vi "K-Means Clusters 1D.vi"() -> ()   [LabVIEW 2018]
uses:
  <vilib>/Analysis/5stat.llb/RMS (DBL).vi
  <vilib>/Analysis/baseanly.llb/Mean (DBL).vi
  <vilib>/Analysis/NI_AALBase.lvlib
  <vilib>/Analysis/NI_AALPro.lvlib
panel:
  out "Statistics":cluster{"mean":dbl, "rms":dbl, "median":dbl}[](array[cluster])
  out "Iteration":i32
  in  "Abs Max":dbl=100.0
  in  "Abs Min":dbl=-100.0
  in  "Normalize":T1(ring)
  out "K-Means Clusters":cluster{dbl[]}[](array[cluster])
  out "K-Means Graph":cluster{dbl[]}[](graph)
  in  "Num of Clusters (5)":i32=5
  in  "Data Set":dbl[](array[numeric])=[11.0, 12.0, 13.0, 21.0, 22.0, 23.0, 31.0, 32.0, 33.0, 41.0, 42.0, 43.0, 51.0, 52.0, 53.0, 16.0, 17.0, 18.0, 16.0]
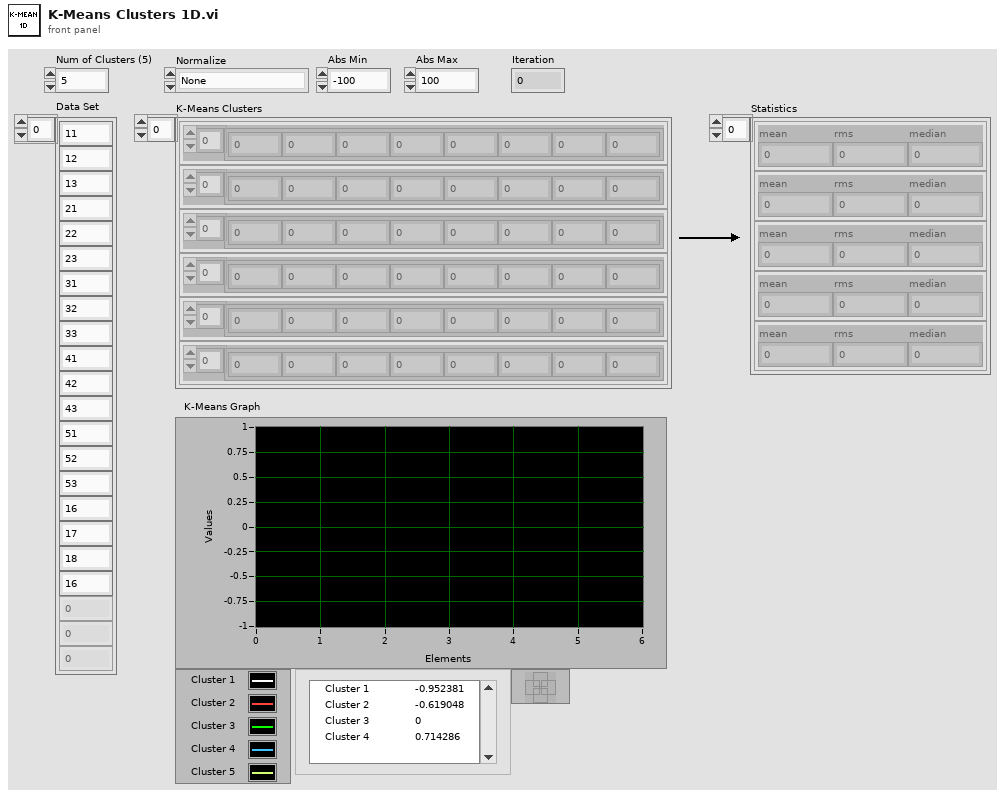
[diagram p1: front panel]
types:
  T1 = enum16{"None", "Data Set Min..Max -> 0..1", "Data Set Min..Max -> -1..1", "Absolute Min..Max -> 0..1", "Absolute Min..Max -> -1..1"}
  T2 = cluster{"mean":dbl, "rms value":dbl, "median":dbl}
  T3 = cluster{"Name":string, "Color":u32, "Style":u8, "Point Style":u8, "Name Visible":bool, "Allow Drag":bool, "Cursor Mode":u32, "Plot":i32, "Index":i32, "Position":cluster{"X":dbl, "Y":dbl}, "X Scale":u32, "Y Scale":u32, "Watch Plots":i32[], "Watch All Plots":bool, "Plot Area":i32, "Label Offset":cluster{"X":dbl, "Y":dbl}}
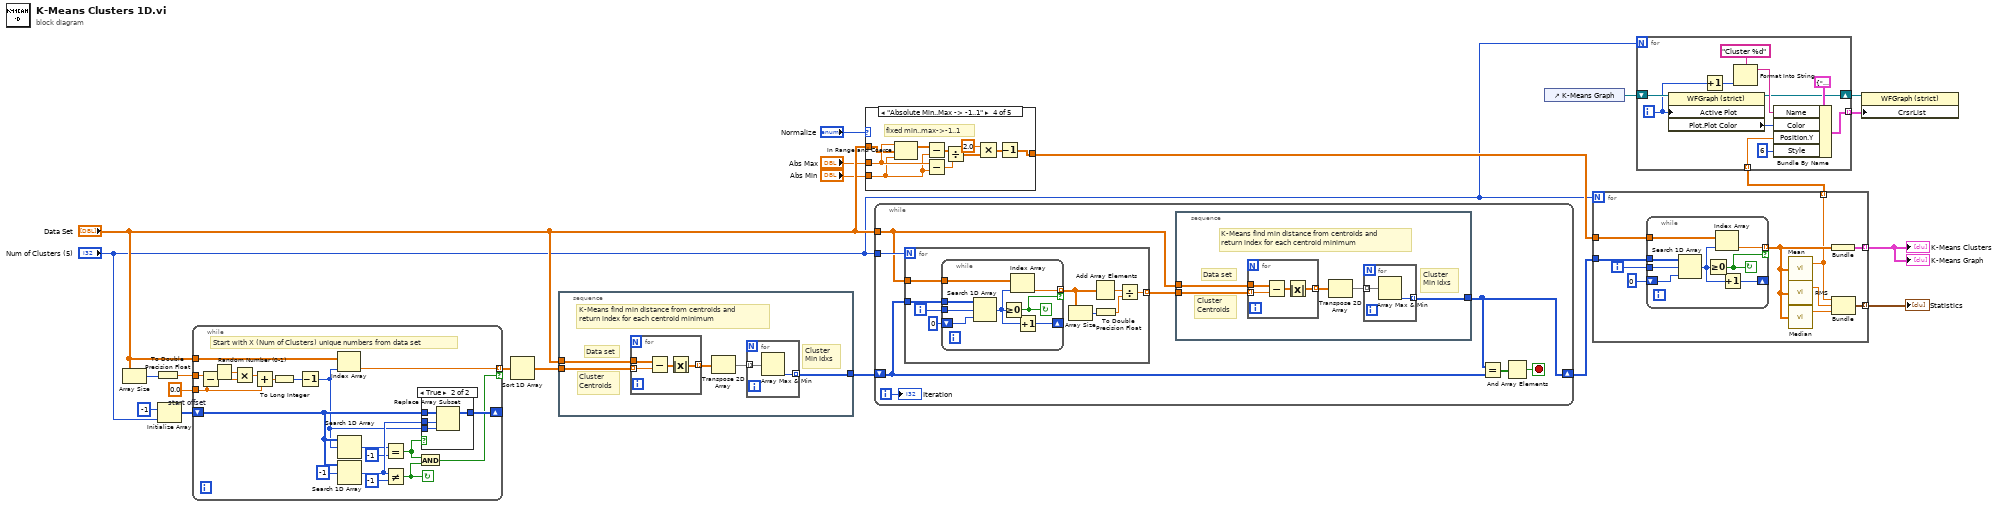
[diagram p0: block diagram]
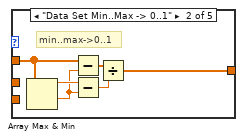
[diagram p4: hidden frame]
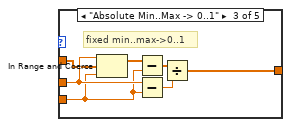
[diagram p5: hidden frame]
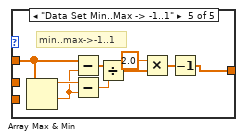
[diagram p6: hidden frame]
diagram:
  w14 = 0.0  # start offset
  n1 = Array Size(array="Data Set") -> (size(s)=w21:i32)
  n2 = To Double Precision Float(number=w21) -> (double precision float=w15:dbl)
  n3 = Initialize Array(-1 ("32bit integer"), "Num of Clusters (5)") -> (w19:i32[])
  n4 = while {
    tunnel: w15 -> [w38]
    tunnel: "Data Set" -> [w36]
    tunnel: [w35] -> w18 mode=indexing if=w24
    shift-right: [w32] -> _
    shift-left: w19 -> [w30]
    tunnel: w14 -> [w22]
    stop <- w25 continue-if-true
    # "Start with X (Num of Clusters) unique numbers from data set"
    n5 = Subtract(x=w38, y=w22) -> (x-y=w41:dbl)
    n6 = Random Number (0-1)() -> (number: 0 to 1=w40:dbl)
    n7 = Multiply(x=w40, y=w41) -> (x*y=w39:dbl)
    n8 = Add(x=w39, y=w22) -> (x+y=w37:dbl)
    n9 = To Long Integer(number=w37) -> (32bit integer=w29:i32)
    n10 = Decrement(x=w29) -> (x-1=w23:i32)
    n11 = Index Array(array=w36, index=w23) -> (element=w35:dbl)
    n12 = Search 1D Array(1D array=w30, element=w23) -> (index of element=w27:i32)  [unwired: 1 in]
    n13 = Search 1D Array(1D array=w30, element=-1) -> (index of element=w31:i32)  [unwired: 1 in]
    n14 = Equal?(x=w27, y=-1) -> (x = y?=w26:bool)
    n15 = Not Equal?(x=w31, y=-1) -> (x != y?=w25:bool)
    n16 = And(x=w26, y=w25) -> (x .and. y?=w24:bool)
    n17 = case shown="True" w26 {
      tunnel: w30 -> [w42 w46]
      tunnel: w23 -> [_ w44]
      tunnel: [w42 w45] -> w32
      tunnel: w31 -> [_ w43]
      frame False {
      }
      frame True {
        n18 = Replace Array Subset(array=w46, new element=w44, index=w43) -> (w45:i32[])
      }
    }
  }
  n19 = Sort 1D Array(array=w18) -> (sorted array=w17:dbl[])
  n20 = stacked-sequence {
    tunnel: [w47] -> w16
    tunnel: w17 -> [w51]
    tunnel: "Data Set" -> [w50]
    frame #0 {
      # "Cluster\nMin Idxs"
      # "K-Means find min distance from centroids and \nreturn index for each centroid minimum"
      # "Cluster\nCentroids"
      # "Data set"
      n21 = for {
        tunnel: w51 -> [w54] mode=indexing
        tunnel: w50 -> [w55]
        tunnel: [w52] -> w49 mode=indexing
        n22 = Subtract(x=w55, y=w54) -> (x-y=w53:dbl[])
        n23 = Absolute Value(x=w53) -> (abs(x)=w52:dbl[])
      }
      n24 = Transpose 2D Array(2D array=w49) -> (transposed array=w48:dbl[][])
      n25 = for {
        tunnel: w48 -> [w57] mode=indexing
        tunnel: [w56] -> w47 mode=indexing
        n26 = Array Max & Min(array=w57) -> (min index (indices)=w56:i32)  [unwired: 3 out]
      }
    }
  }
  n27 = case shown="\"Absolute Min..Max -> -1..1\"" "Normalize" {
    tunnel: "Data Set" -> [w58 w60 w65 w76 w86]
    tunnel: [w58 w59 w69 w73 w82] -> w11
    tunnel: "Abs Max" -> [_ _ w68 w79 _]
    tunnel: "Abs Min" -> [_ _ w67 w78 _]
    frame "None" {
    }
    frame "Data Set Min..Max -> 0..1" {
      # "min..max->0..1"
      n28 = Array Max & Min(array=w60) -> (max value=w64:dbl, min value=w63:dbl)  [unwired: 2 out]
      n29 = Subtract(x=w60, y=w63) -> (x-y=w62:dbl[])
      n30 = Subtract(x=w64, y=w63) -> (x-y=w61:dbl)
      n31 = Divide(x=w62, y=w61) -> (x/y=w59:dbl[])
    }
    frame "Absolute Min..Max -> 0..1" {
      # "fixed min..max->0..1"
      n32 = In Range and Coerce(upper limit=w68, x=w65, lower limit=w67) -> (coerced(x)=w66:dbl[])  [unwired: 1 out]
      n33 = Subtract(x=w66, y=w67) -> (x-y=w71:dbl[])
      n34 = Subtract(x=w68, y=w67) -> (x-y=w70:dbl)
      n35 = Divide(x=w71, y=w70) -> (x/y=w69:dbl[])
    }
    frame "Absolute Min..Max -> -1..1" {
      # "fixed min..max->-1..1"
      n36 = In Range and Coerce(upper limit=w79, x=w76, lower limit=w78) -> (coerced(x)=w77:dbl[])  [unwired: 1 out]
      n37 = Subtract(x=w77, y=w78) -> (x-y=w81:dbl[])
      n38 = Subtract(x=w79, y=w78) -> (x-y=w80:dbl)
      n39 = Divide(x=w81, y=w80) -> (x/y=w74:dbl[])
      n40 = Multiply(x=2.0 ("DBL"), y=w74) -> (x*y=w75:dbl[])
      n41 = Decrement(x=w75) -> (x-1=w73:dbl[])
    }
    frame "Data Set Min..Max -> -1..1" {
      # "min..max->-1..1"
      n42 = Array Max & Min(array=w86) -> (max value=w90:dbl, min value=w89:dbl)  [unwired: 2 out]
      n43 = Subtract(x=w86, y=w89) -> (x-y=w88:dbl[])
      n44 = Subtract(x=w90, y=w89) -> (x-y=w87:dbl)
      n45 = Divide(x=w88, y=w87) -> (x/y=w83:dbl[])
      n46 = Multiply(x=2.0, y=w83) -> (x*y=w84:dbl[])
      n47 = Decrement(x=w84) -> (x-1=w82:dbl[])
    }
  }
  n48 = while {
    tunnel: "Data Set" -> [w94]
    shift-right: [w92] -> w7
    shift-left: w16 -> [w98]
    tunnel: "Num of Clusters (5)" -> [w95]
    i -> [w91]
    stop <- w97 stop-if-true
    n49 = for {
      N: w95 -> [_]
      tunnel: w98 -> [w114]
      tunnel: w94 -> [w111]
      tunnel: [w116] -> w93 mode=indexing
      i -> [w113]
      n50 = while {
        tunnel: w114 -> [w126]
        tunnel: w113 -> [w125]
        shift-right: [w119] -> _
        shift-left: 0 ("start index (0)") -> [w124]
        tunnel: w111 -> [w122]
        tunnel: [w121] -> w110 mode=indexing if=w120
        stop <- w120 continue-if-true
        n51 = Search 1D Array(1D array=w126, element=w125, start index (0)=w124) -> (index of element=w123:i32)
        n52 = Greater Or Equal To 0?(x=w123) -> (x >= 0?=w120:bool)
        n53 = Index Array(array=w122, index=w123) -> (element=w121:dbl)
        n54 = Increment(x=w123) -> (x+1=w119:i32)
      }
      n55 = Array Size(array=w110) -> (size(s)=w117:i32)
      n56 = Add Array Elements(numeric array=w110) -> (sum=w118:dbl)
      n57 = To Double Precision Float(number=w117) -> (double precision float=w115:dbl)
      n58 = Divide(x=w118, y=w115) -> (x/y=w116:dbl)
    }
    n59 = stacked-sequence {
      tunnel: [w99] -> w92
      tunnel: w93 -> [w103]
      tunnel: w94 -> [w102]
      frame #0 {
        # "Cluster\nMin Idxs"
        # "K-Means find min distance from centroids and \nreturn index for each centroid minimum"
        # "Cluster\nCentroids"
        # "Data set"
        n60 = for {
          tunnel: w103 -> [w106] mode=indexing
          tunnel: w102 -> [w107]
          tunnel: [w104] -> w101 mode=indexing
          n61 = Subtract(x=w107, y=w106) -> (x-y=w105:dbl[])
          n62 = Absolute Value(x=w105) -> (abs(x)=w104:dbl[])
        }
        n63 = Transpose 2D Array(2D array=w101) -> (transposed array=w100:dbl[][])
        n64 = for {
          tunnel: w100 -> [w109] mode=indexing
          tunnel: [w108] -> w99 mode=indexing
          n65 = Array Max & Min(array=w109) -> (min index (indices)=w108:i32)  [unwired: 3 out]
        }
      }
    }
    n66 = Equal?(x=w92, y=w98) -> (x = y?=w96:bool[])
    n67 = And Array Elements(Boolean array=w96) -> (logical AND=w97:bool)
    "Iteration" <- w91
  }
  n68 = control-ref of="K-Means Graph"() -> (w2:refnum<vi>)
  n69 = for {
    N: "Num of Clusters (5)" -> [_]
    tunnel: w7 -> [w135]
    tunnel: w11 -> [w136]
    tunnel: [w133] -> w13 mode=indexing
    tunnel: [w128] -> w6 mode=indexing
    tunnel: [w127] -> w4 mode=indexing
    i -> [w132]
    n70 = while {
      tunnel: w135 -> [w144]
      tunnel: w132 -> [w143]
      shift-right: [w137] -> _
      shift-left: 0 ("start index (0)") -> [w142]
      tunnel: w136 -> [w140]
      tunnel: [w139] -> w130 mode=indexing if=w138
      stop <- w138 continue-if-true
      n71 = Search 1D Array(1D array=w144, element=w143, start index (0)=w142) -> (index of element=w141:i32)
      n72 = Greater Or Equal To 0?(x=w141) -> (x >= 0?=w138:bool)
      n73 = Index Array(array=w140, index=w141) -> (element=w139:dbl)
      n74 = Increment(x=w141) -> (x+1=w137:i32)
    }
    n75 = call-poly <vilib>:"Mean.vi"("X"=w130) -> ("mean"=w127:dbl)  [unwired: 1 out]
    n76 = call-poly <vilib>:"RMS.vi"("X"=w130) -> ("rms value"=w131:dbl)  [unwired: 1 out]
    n77 = call <vilib>:"Median.vi"("X"=w130) -> ("median"=w129:dbl)  [unwired: 1 out]
    n78 = Bundle(w130) -> (w133:cluster{dbl[]})  [unwired: 1 in]
    n79 = Bundle("mean"=w127, "rms value"=w131, "median"=w129) -> (w128:T2)  [unwired: 1 in]
  }
  "K-Means Graph" <- w13
  "K-Means Clusters" <- w13
  "Statistics" <- w6
  n80 = for {
    N: "Num of Clusters (5)" -> [_]
    tunnel: w4 -> [w153] mode=indexing
    tunnel: [w152] -> w3 mode=indexing
    shift-right: [w145] -> w1
    shift-left: w2 -> [w155]
    i -> [w151]
    n81 = property class="WFGraph (strict)"(reference=w155, "Active Plot"=w151) -> (reference out=w145:refnum<vi>, "Plot.Plot Color"=w147:u32)  [unwired: 1 in, 1 out]
    n82 = Increment(x=w151) -> (x+1=w150:i32)
    n83 = Format Into String(format string="Cluster %d", w150) -> (resulting string=w148:string)  [unwired: 2 in, 1 out]
    n84 = Bundle By Name(cluster=T3 {"Name"="", "Color"=0, "Style"=0, "Point Style"=0, "Name Visible"=FALSE, "Allow Drag"=FALSE, "Cursor Mode"=0, "Plot"=0, "Index"=0, "Position"={"X"=0.0, "Y"=0.0}, "X Scale"=0, "Y Scale"=0, "Watch Plots"=[], "Watch All Plots"=FALSE, "Plot Area"=0, "Label Offset"={"X"=0.0, "Y"=0.0}}, "Name"=w148, "Color"=w147, "Position.Y"=w153, "Style"=u8 6) -> (w152:T3)
  }
  n85 = property on="Property Node" class="WFGraph (strict)"(reference=w1, "CrsrList"=w3) -> ()  [unwired: 1 in, 2 out]
